vi "Event Current Context I32.vi"(8 "error in":errorcluster, 11 "Context in":refnum<class "Context.lvclass">) -> (0 "error out":errorcluster, 3 "Context out":refnum<class "Context.lvclass">)   [LabVIEW 2021, in "Context.lvlib" / "Context.lvclass"]
uses:
  Context.lvclass
  Context.lvclass/Context.ctl
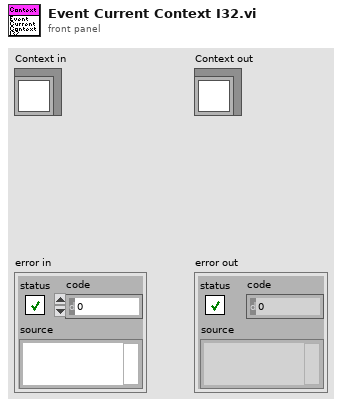
[diagram p1: front panel]
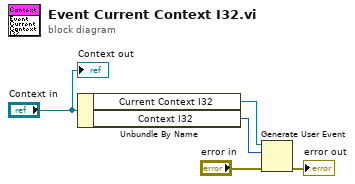
[diagram p0: block diagram]
diagram:
  n1 = Unbundle By Name("Context in") -> ("Current Context I32"=w4:refnum<user-event>, "Context I32"=w1:i32)
  n2 = Generate User Event(user event=w4, event data cluster=w1, error in="error in") -> (error out=→"error out":errorcluster)  [unwired: 1 in, 1 out]
  "Context out" <- "Context in"
